vi "SetUpInstruments.vi"(8 "ErrorIn(No Error)":errorcluster caption="entrée d'erreur (pas d'erreur)", 11 "Experiment.lvclass":refnum<class "Experiment.lvclass">) -> (0 "sortie d'erreur":errorcluster, 3 "Experiment.lvclass Out":refnum<class "Experiment.lvclass">)   [LabVIEW 2019, in "Experiment.lvclass"]
uses:
  Experiment.lvclass
  LoadInstr.ctl
  SetUpInstrStates.ctl
  Experiment.lvclass/Experiment.ctl
  DevicesClass/BaseDevice/BaseDevice.lvclass
panel:
  out "Classindex":i32
  in  "ScanRes":bool=TRUE
  in  "Modify":bool
  in  "Remove":bool
  in  "LoadInstr":T1
  in  "LoadedDev":string(tree)
  in  "AvailableDev":string(tree)
  in  "stop":bool
  in  "Add Instrument":bool
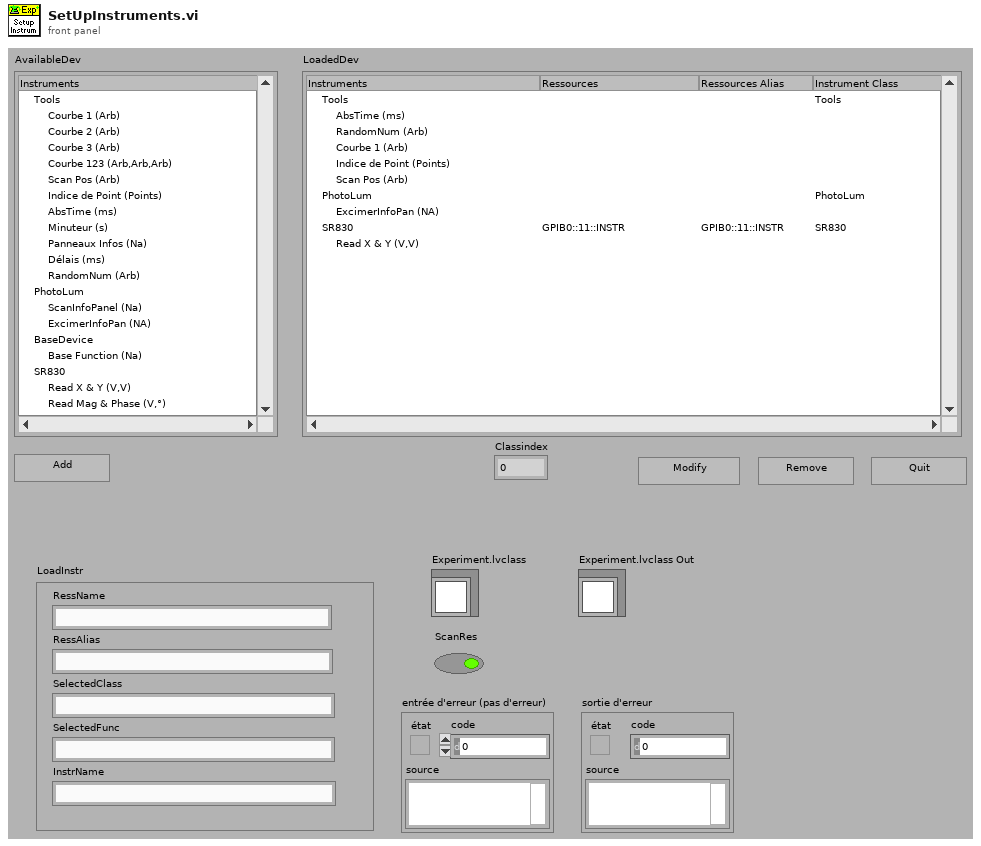
[diagram p1: front panel]
types:
  T1 = typedef "LoadInstr.ctl" = cluster{"SelectedClass":string, "SelectedFunc":string, "InstrName":string, "RessAlias":string, "RessName":string}
  T2 = typedef "SetUpInstrStates.ctl" = enum16{"InitCtrls", "InitProg", "CheckIfInstr", "AddNonInstrFunc", "InstrClassExist?", "AddFuncNewInstr", "AddFuncExInstr", "FuncToWhichInstr?", "ConfirmUnload?", "Unload Instrument", "Unload Function", "ModifyInstr", "Stop", "Error"}
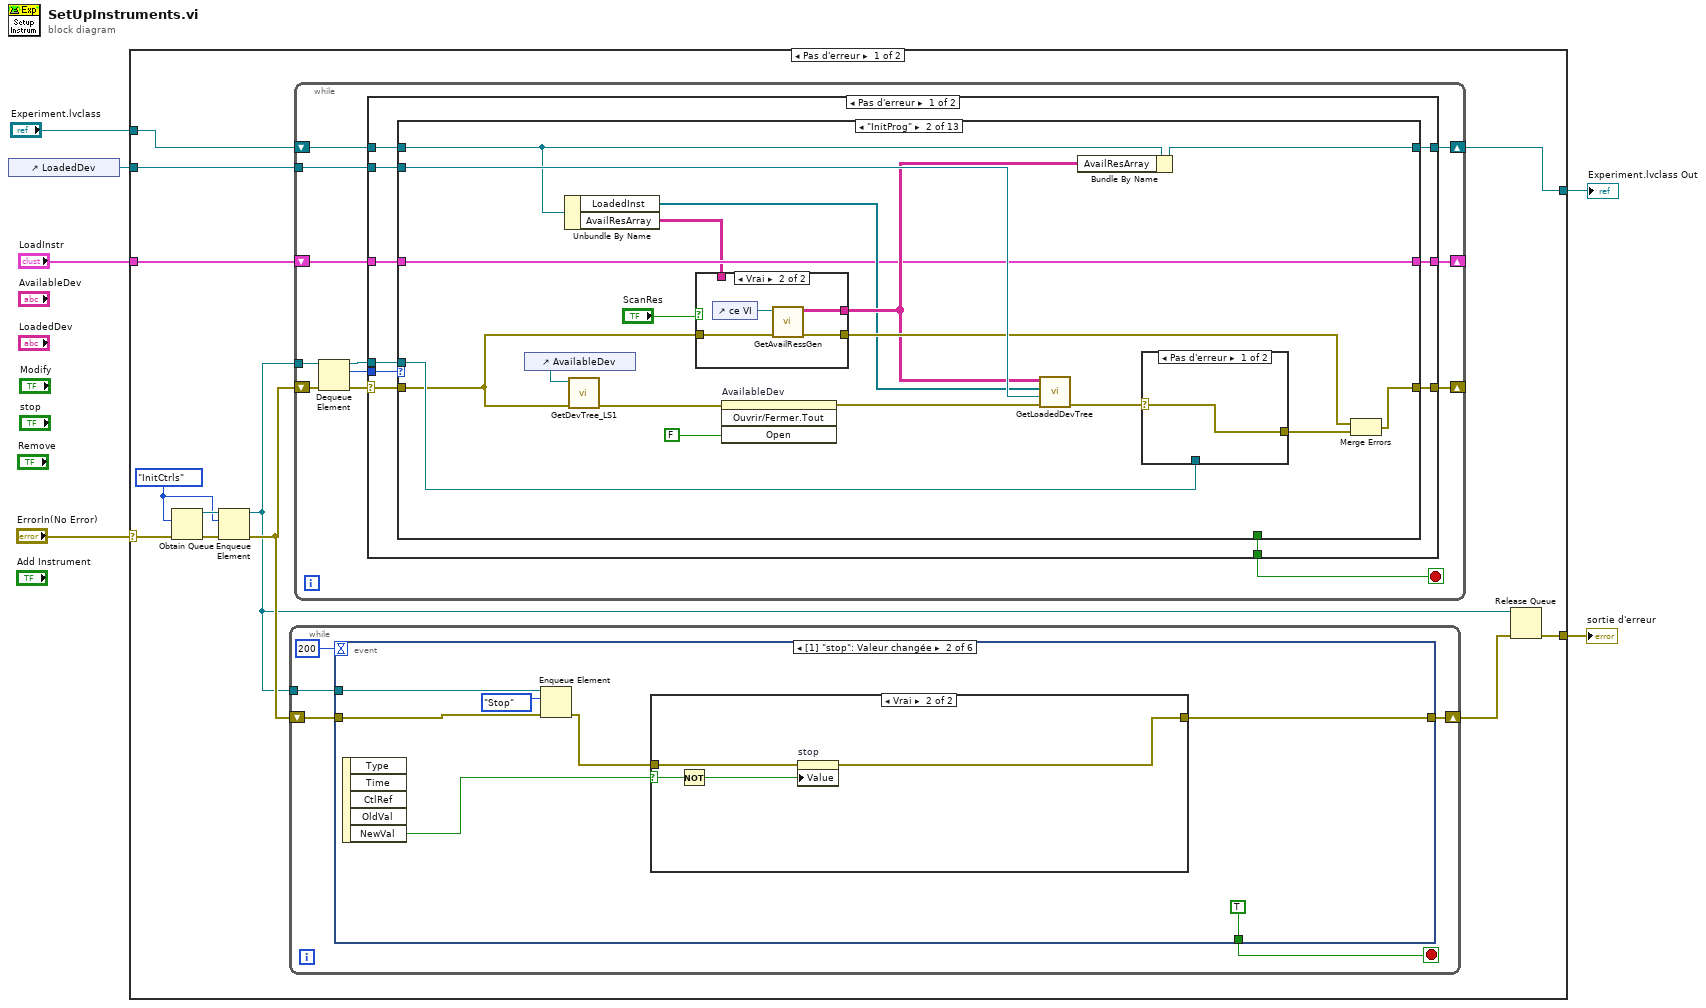
[diagram p0: block diagram]
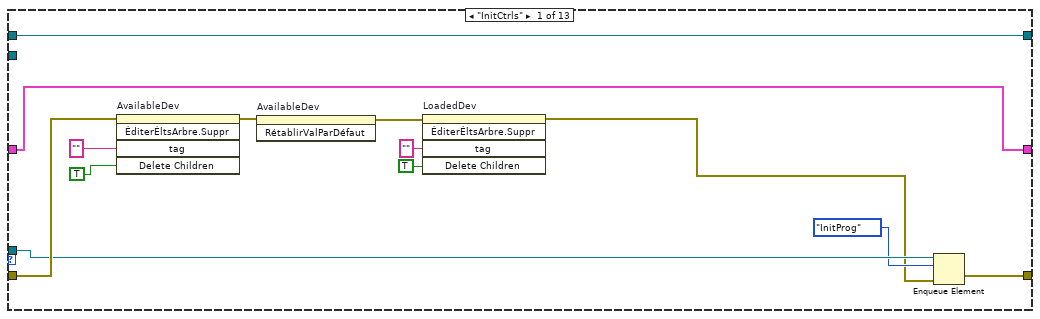
[diagram p2: hidden frame]
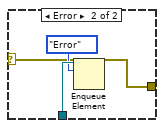
[diagram p4: hidden frame]
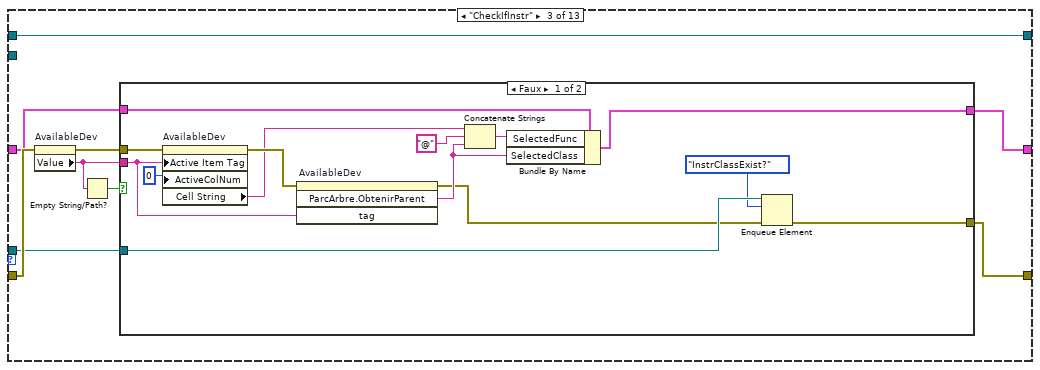
[diagram p5: hidden frame]
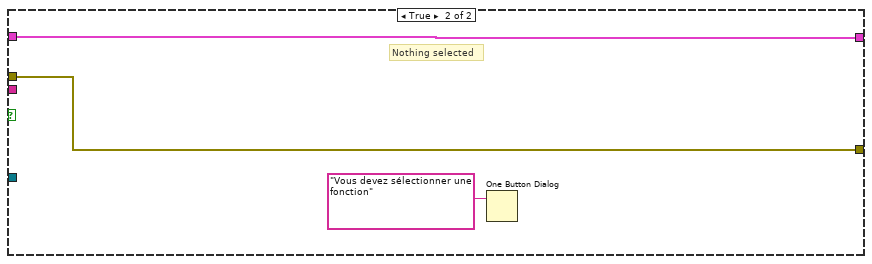
[diagram p6: hidden frame]
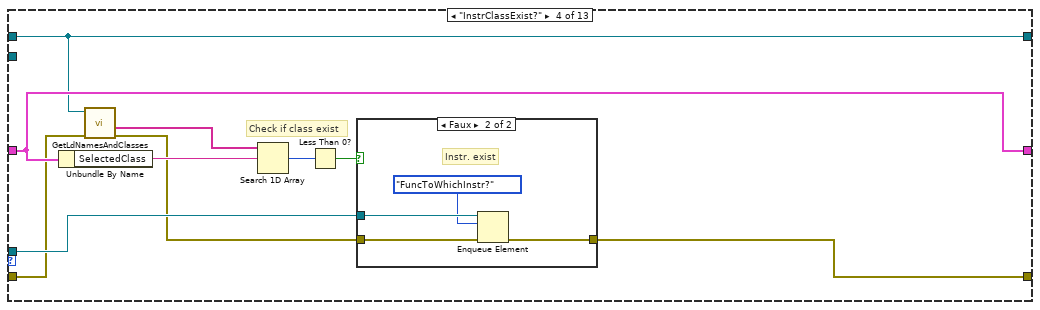
[diagram p7: hidden frame]
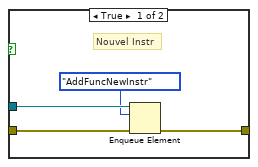
[diagram p8: hidden frame]
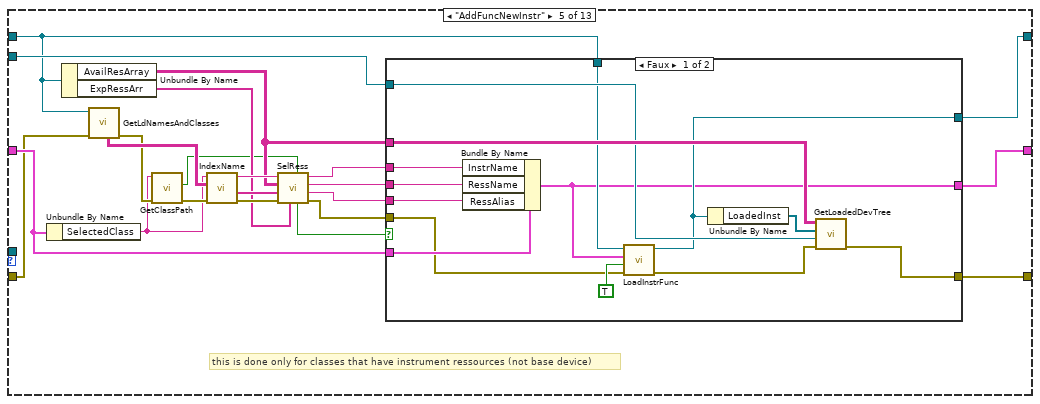
[diagram p9: hidden frame]
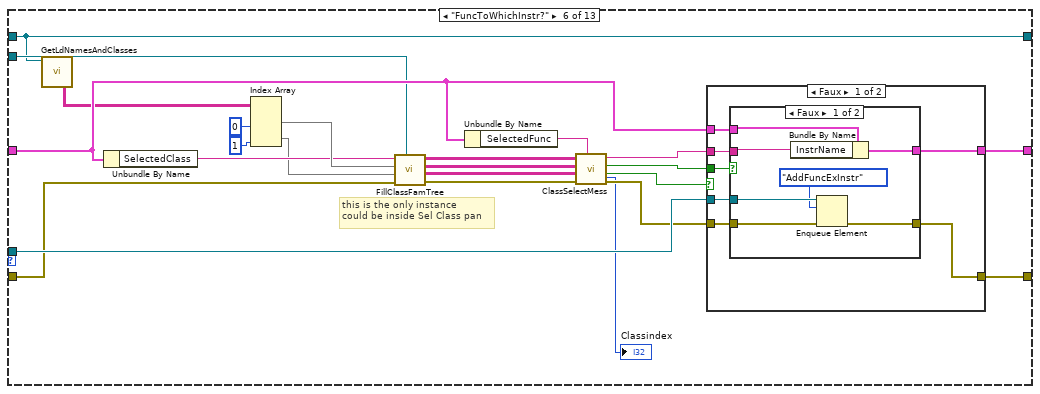
[diagram p11: hidden frame]
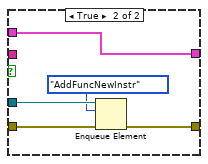
[diagram p12: hidden frame]
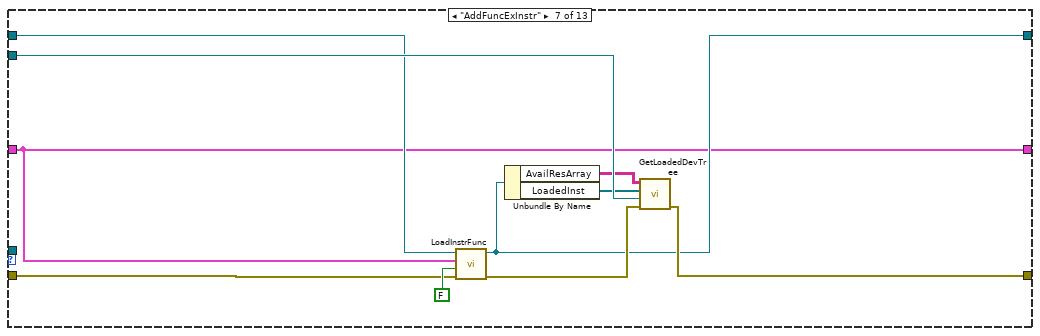
[diagram p14: hidden frame]
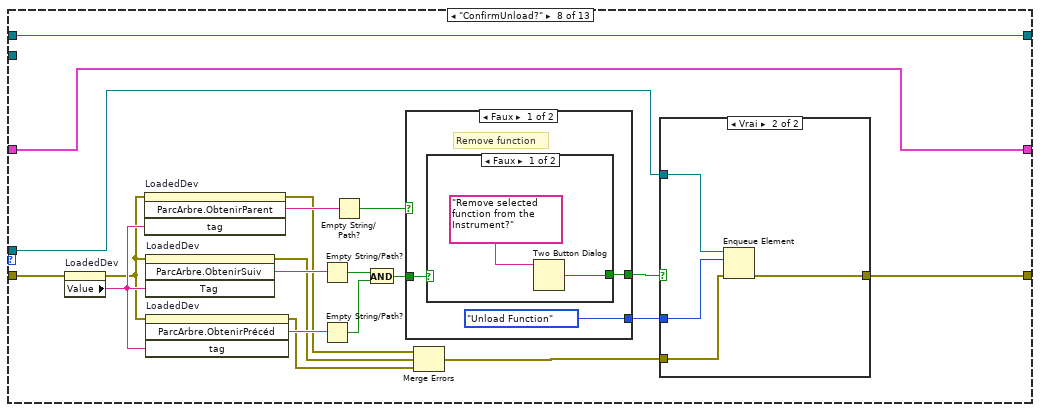
[diagram p15: hidden frame]
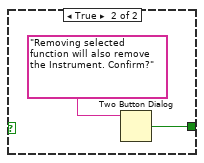
[diagram p17: hidden frame]
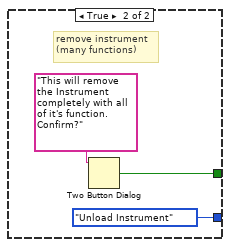
[diagram p18: hidden frame]
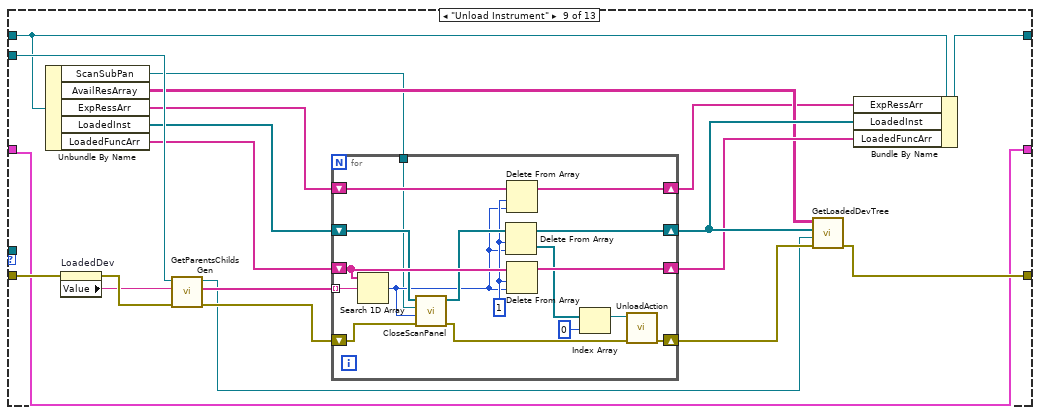
[diagram p19: hidden frame]
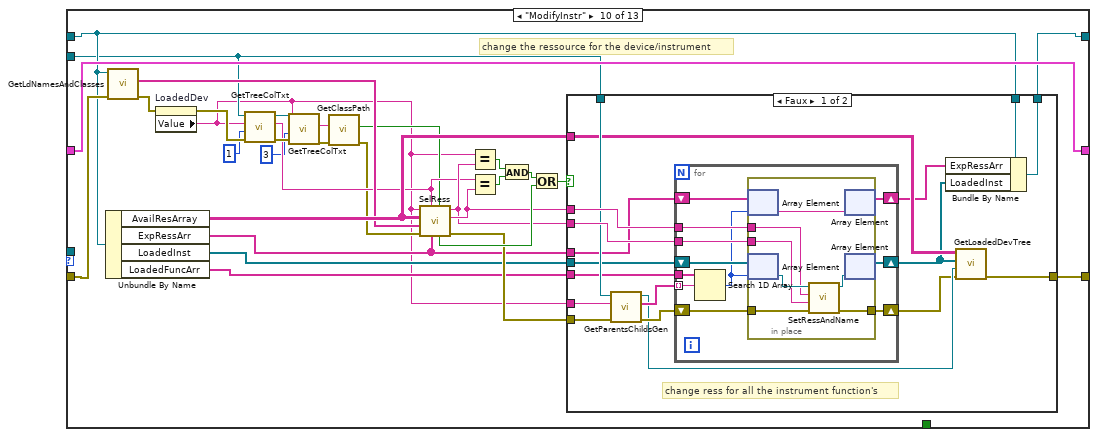
[diagram p20: hidden frame]
diagram:
  n1 = control-ref of="LoadedDev"() -> (w4:refnum<vi>)
  n2 = case shown="Pas d'erreur" "ErrorIn(No Error)" {
    selector: "ErrorIn(No Error)" -> [w9 w479]
    tunnel: "LoadInstr" -> [w14 _]
    tunnel: w4 -> [w13 _]
    tunnel: [w10 w479] -> w3
    tunnel: "Experiment.lvclass" -> [w8 w478]
    tunnel: [w7 w478] -> w1
    frame No Error {
      w16 = SetUpInstrStates."InitCtrls" ("Énum")
      n3 = Obtain Queue(element data type=w16, error in (no error)=w9) -> (queue out=w18:refnum<queue>, error out=w17:errorcluster)  [unwired: 3 in, 1 out]
      n4 = Enqueue Element(queue=w18, element=w16, error in (no error)=w17) -> (queue out=w11:refnum<queue>, error out=w15:errorcluster)  [unwired: 1 in, 1 out]
      n5 = while {
        shift-right: [w397] -> w12
        shift-left: w15 -> [w400]
        tunnel: w11 -> [w398]
        stop <- w399 stop-if-true
        n6 = event shown="[1] \"stop\": Valeur changée" {
          selector: _ -> [_ _ _ _ _ _]
          dyn-events: _ -> [_ _ _ _ _ _]
          timeout: 200 -> [_ _ _ _ _ _]
          tunnel: w400 -> [_ w407 w420 w424 w434 w439]
          tunnel: [_ TRUE ("stop") _ TRUE ("stop") _ _] -> w399
          tunnel: w398 -> [_ w408 w419 w425 w433 w437]
          tunnel: [_ w402 w417 w423 w431 w438] -> w397
          event Timeout {
            n7 = event-data() -> ()  [unwired: 1 in, 2 out]
          }
          event "stop": Value Change {
            n8 = event-data() -> ("NewVal"=w404:bool)  [unwired: 1 in, 4 out]
            n9 = Enqueue Element(queue=w408, element=SetUpInstrStates."Stop" ("élément"), error in (no error)=w407) -> (error out=w403:errorcluster)  [unwired: 1 in, 2 out]
            n10 = case shown="Vrai" w404 {
              selector: w404 -> [_ w413]
              tunnel: w403 -> [w409 w411]
              tunnel: [w409 w410] -> w402
              frame False {
              }
              frame True {
                n11 = Not(x=w413) -> (.not. x?=w412:bool)
                n12 = property on="stop" class="Bool (strict)"(error in=w411, "Value"=w412) -> (error out=w410:errorcluster)  [unwired: 1 in, 1 out]
              }
            }
          }
          event "Add Instrument": Value Change {
            n13 = event-data() -> ("NewVal"=w416:bool)  [unwired: 1 in, 4 out]
            n14 = Wait (ms)(milliseconds to wait=u32 200 ("attente (ms)")) -> (millisecond timer value=w414:u32)
            n15 = Enqueue Element(queue=w419, element=SetUpInstrStates."CheckIfInstr" ("élément"), error in (no error)=w420) -> (error out=w417:errorcluster)  [unwired: 1 in, 2 out]
            n16 = case shown="Vrai" w416 {
              selector: w416 -> [_ w422]
              tunnel: w414 -> [_ _]
              frame False {
              }
              frame True {
                n17 = Not(x=w422) -> (.not. x?=w421:bool)
                n18 = property on="Add Instrument" class="Bool (strict)"("Value"=w421) -> ()  [unwired: 2 in, 2 out]
              }
            }
          }
          event Panel Close {
            n19 = event-data() -> ()  [unwired: 1 in, 4 out]
            n20 = Enqueue Element(queue=w425, element=SetUpInstrStates."Stop" ("élément"), error in (no error)=w424) -> (error out=w423:errorcluster)  [unwired: 1 in, 2 out]
          }
          event "Remove": Value Change {
            n21 = event-data() -> ("NewVal"=w430:bool)  [unwired: 1 in, 4 out]
            n22 = Wait (ms)(milliseconds to wait=u32 200 ("attente (ms)")) -> (millisecond timer value=w428:u32)
            n23 = Enqueue Element(queue=w433, element=SetUpInstrStates."ConfirmUnload?" ("élément"), error in (no error)=w434) -> (error out=w431:errorcluster)  [unwired: 1 in, 2 out]
            n24 = case shown="Vrai" w430 {
              selector: w430 -> [_ w436]
              tunnel: w428 -> [_ _]
              frame False {
              }
              frame True {
                n25 = Not(x=w436) -> (.not. x?=w435:bool)
                n26 = property on="Remove" class="Bool (strict)"("Value"=w435) -> ()  [unwired: 2 in, 2 out]
              }
            }
          }
          event "Modify": Value Change {
            n27 = event-data() -> ("NewVal"=w440:bool)  [unwired: 1 in]
            n28 = case shown="Vrai" w440 {
              tunnel: w439 -> [w441 w447]
              tunnel: [w441 w445] -> w438
              tunnel: w437 -> [_ w443]
              frame False {
              }
              frame True {
                n29 = property on="LoadedDev" class="Arbre (strict)"(error in=w447) -> (error out=w454:errorcluster, "Value"=w442:string)  [unwired: 1 in, 1 out]
                n30 = invoke on="LoadedDev" class="Arbre (strict)" method="ParcArbre.ObtenirEnfant"(error in=w454, "Tag"=w442) -> (error out=w451:errorcluster, "Navigate Tree:Get Child"=w456:string)  [unwired: 2 in, 2 out]
                n31 = invoke on="LoadedDev" class="Arbre (strict)" method="ParcArbre.ObtenirParent"(error in=w454, "tag"=w442) -> (error out=w452:errorcluster, "Navigate Tree:Get Parent"=w453:string)  [unwired: 2 in, 2 out]
                n32 = Merge Errors(w451, w452) -> (w450:errorcluster)
                n33 = Empty String/Path?(string/path=w456) -> (empty?=w455:bool)
                n34 = case shown="Faux" w455 {
                  tunnel: w453 -> [_ w469]
                  tunnel: w450 -> [w463 w464]
                  tunnel: [TRUE w471] -> w449
                  tunnel: [w463 w470] -> w448
                  tunnel: w442 -> [_ _]
                  frame False {
                    # "instrument selected"
                  }
                  frame True {
                    # "func selected"
                    n35 = Format Into String(format string="This will modify parent instrument %s and all of it's functions! Continue? " ("message"), error in=w464, w469) -> (resulting string=w467:string, error out=w466:errorcluster)  [unwired: 1 in]
                    n36 = Two Button Dialog(message=w467) -> (T button?=w465:bool)  [unwired: 2 in]
                    n37 = case shown="Vrai" w465 {
                      selector: w465 -> [w473 w475]
                      tunnel: w469 -> [_ w477]
                      tunnel: w466 -> [w472 w476]
                      tunnel: [w473 w475] -> w471
                      tunnel: [w472 w474] -> w470
                      frame False {
                      }
                      frame True {
                        n38 = property on="LoadedDev" class="Arbre (strict)"(error in=w476, "Value"=w477) -> (error out=w474:errorcluster)  [unwired: 1 in, 1 out]
                      }
                    }
                  }
                }
                n39 = case shown="Vrai" w449 {
                  tunnel: w448 -> [w457 w460]
                  tunnel: [w457 w459] -> w446
                  tunnel: w443 -> [_ w458]
                  frame False {
                  }
                  frame True {
                    n40 = Enqueue Element(queue=w458, element=SetUpInstrStates."ModifyInstr" ("élément"), error in (no error)=w460) -> (error out=w459:errorcluster)  [unwired: 1 in, 2 out]
                  }
                }
                n41 = property on="Modify" class="Bool (strict)"(error in=w446, "Value"=FALSE ("Modify")) -> (error out=w445:errorcluster)  [unwired: 1 in, 1 out]
              }
            }
          }
        }
      }
      n42 = while {
        tunnel: w11 -> [w27]
        shift-right: [w24] -> _
        shift-left: w15 -> [w30]
        shift-right: [w21] -> _
        shift-left: w14 -> [w23]
        tunnel: w13 -> [w22]
        shift-right: [w19] -> w7
        shift-left: w8 -> [w20]
        stop <- w26 stop-if-true
        n43 = Dequeue Element(queue=w27, error in (no error)=w30) -> (queue out=w25:refnum<queue>, element=w28:T2, error out=w29:errorcluster)  [unwired: 1 in, 1 out]
        n44 = case shown="Pas d'erreur" w29 {
          selector: w29 -> [w38 w395]
          tunnel: w28 -> [w40 _]
          tunnel: [w39 FALSE] -> w26
          tunnel: w25 -> [w37 _]
          tunnel: [w36 w391] -> w24
          tunnel: w23 -> [w35 w394]
          tunnel: w22 -> [w34 _]
          tunnel: [w33 w394] -> w21
          tunnel: w20 -> [w32 w393]
          tunnel: [w31 w393] -> w19
          frame No Error {
            n45 = case shown="\"InitProg\"" w40 {
              tunnel: [_ _ _ _ _ _ _ _ _ _ _ TRUE TRUE] -> w39
              tunnel: w38 -> [w50 w56 w90 w109 w130 w175 w211 w238 w273 w307 w382 w384 w388]
              tunnel: w37 -> [w49 w67 w89 w116 _ w181 _ w223 _ _ _ _ _]
              tunnel: [w48 w66 w88 w113 w145 w180 w215 w221 w272 w317 w379 w384 w388] -> w36
              tunnel: w35 -> [w46 w57 w87 w114 w139 w185 w209 w220 w255 w308 w361 w385 w389]
              tunnel: w34 -> [_ w63 _ _ w138 w174 w217 _ w270 w301 w380 _ _]
              tunnel: [w46 w57 w86 w114 w137 w183 w209 w220 w255 w308 w361 w385 w389] -> w33
              tunnel: w32 -> [w45 w59 w85 w111 w131 w167 w214 w219 w265 w305 w373 w383 w387]
              tunnel: [w45 w61 w85 w111 w135 w167 w213 w219 w262 w304 w372 w383 w387] -> w31
              frame "InitCtrls" {
                n46 = invoke on="AvailableDev" class="Arbre (strict)" method="ÉditerÉltsArbre.Suppr"(error in=w50, "tag"="" ("Tag"), "Delete Children"=TRUE ("Supprimer les enfants ?")) -> (error out=w51:errorcluster)  [unwired: 2 in, 4 out]
                n47 = invoke on="AvailableDev" class="Arbre (strict)" method="RétablirValParDéfaut"(error in=w51) -> (error out=w44:errorcluster)  [unwired: 2 in, 2 out]
                n48 = invoke on="LoadedDev" class="Arbre (strict)" method="ÉditerÉltsArbre.Suppr"(error in=w44, "tag"="" ("Tag"), "Delete Children"=TRUE ("Supprimer les enfants ?")) -> (error out=w43:errorcluster)  [unwired: 2 in, 4 out]
                n49 = Enqueue Element(queue=w49, element=SetUpInstrStates."InitProg" ("élément"), error in (no error)=w43) -> (error out=w48:errorcluster)  [unwired: 1 in, 2 out]
              }
              frame "InitProg" {
                n50 = control-ref of="AvailableDev"() -> (w69:refnum<vi>)
                n51 = Unbundle By Name(w59) -> ("LoadedInst"=w58:refnum<class "BaseDevice.lvclass">[], "AvailResArray"=w55:string[][])
                n52 = call "GetDevTree_LS1.vi"("ErrorIn"=w56, "TreeRefIn"=w69) -> ("ErrorOut"=w70:errorcluster)  [unwired: 8 in, 1 out]
                n53 = case shown="Vrai" "ScanRes" {
                  tunnel: [w72 w77] -> w62
                  tunnel: [w73 w76] -> w60
                  tunnel: w56 -> [w72 w75]
                  tunnel: w55 -> [w73 _]
                  frame False {
                  }
                  frame True {
                    n54 = control-ref of="ce VI"() -> (w74:refnum<vi>)
                    n55 = call <userlib>:"GetAvailRessGen.vi"("ErrorIn(No Error)"=w75, "VI reference"=w74) -> ("sortie d'erreur"=w77:errorcluster, "ResArray"=w76:string[][])  [unwired: 8 in]
                  }
                }
                n56 = invoke on="AvailableDev" class="Arbre (strict)" method="Ouvrir/Fermer.Tout"(error in=w70, "Open"=FALSE ("Ouvrir ?")) -> (error out=w71:errorcluster)  [unwired: 2 in, 3 out]
                n57 = call "GetLoadedDevTree.vi"("ErrorIn"=w71, "TreeRefIn"=w63, "LoadedInst"=w58, "AvailRessArray"=w60) -> ("ErrorOut"=w64:errorcluster)  [unwired: 7 in]
                n58 = Bundle By Name(cluster=w59, "AvailResArray"=w60) -> (w61:refnum<class "Experiment.lvclass">)
                n59 = case shown="Pas d'erreur" w64 {
                  selector: w64 -> [w78 w79]
                  tunnel: w67 -> [_ w81]
                  tunnel: [w78 w79] -> w65
                  frame No Error {
                  }
                  frame Error {
                    n60 = Enqueue Element(queue=w81, element=SetUpInstrStates."Error" ("élément")) -> ()  [unwired: 2 in, 3 out]
                  }
                }
                n61 = Merge Errors(w62, w65) -> (w66:errorcluster)
              }
              frame "CheckIfInstr" {
                n62 = property on="AvailableDev" class="Arbre (strict)"(error in=w90) -> (error out=w83:errorcluster, "Value"=w82:string)  [unwired: 1 in, 1 out]
                n63 = Empty String/Path?(string/path=w82) -> (empty?=w84:bool)
                n64 = case shown="Faux" w84 {
                  tunnel: w89 -> [w104 _]
                  tunnel: [w103 w105] -> w88
                  tunnel: w87 -> [w102 w106]
                  tunnel: [w93 w106] -> w86
                  tunnel: w83 -> [w95 w105]
                  tunnel: w82 -> [w94 _]
                  frame False {
                    n65 = property on="AvailableDev" class="Arbre (strict)"(error in=w95, "Active Item Tag"=w94, "ActiveColNum"=0 ("Cellule active : numéro de la colonne active")) -> (error out=w100:errorcluster, "Cell String"=w99:string)  [unwired: 1 in, 1 out]
                    n66 = invoke on="AvailableDev" class="Arbre (strict)" method="ParcArbre.ObtenirParent"(error in=w100, "tag"=w94) -> (error out=w91:errorcluster, "Navigate Tree:Get Parent"=w96:string)  [unwired: 2 in, 2 out]
                    n67 = Concatenate Strings(w99, "@" ("chaîne"), w96) -> (w97:string)
                    n68 = Bundle By Name(cluster=w102, "SelectedFunc"=w97, "SelectedClass"=w96) -> (w93:T1)
                    n69 = Enqueue Element(queue=w104, element=SetUpInstrStates."InstrClassExist?" ("élément"), error in (no error)=w91) -> (error out=w103:errorcluster)  [unwired: 1 in, 2 out]
                  }
                  frame True {
                    # "Nothing selected"
                    n70 = One Button Dialog(message="Vous devez sélectionner une fonction") -> ()  [unwired: 1 in, 1 out]
                  }
                }
              }
              frame "InstrClassExist?" {
                # "Check if class exist"
                n71 = Unbundle By Name(w114) -> ("SelectedClass"=w112:string)
                n72 = call "GetLdNamesAndClasses.vi"("error in (no error)"=w109, "Experiment en entrée"=w111) -> ("error out"=w108:errorcluster, "LdClasses"=w110:string[])  [unwired: 5 in, 3 out]
                n73 = Search 1D Array(1D array=w110, element=w112) -> (index of element=w117:i32)  [unwired: 1 in]
                n74 = Less Than 0?(x=w117) -> (x < 0?=w115:bool)
                n75 = case shown="Faux" w115 {
                  tunnel: w116 -> [w121 w125]
                  tunnel: w108 -> [w119 w123]
                  tunnel: [w118 w122] -> w113
                  frame True {
                    # "Nouvel Instr"
                    n76 = Enqueue Element(queue=w121, element=SetUpInstrStates."AddFuncNewInstr" ("élément"), error in (no error)=w119) -> (error out=w118:errorcluster)  [unwired: 1 in, 2 out]
                  }
                  frame False {
                    # "Instr. exist"
                    n77 = Enqueue Element(queue=w125, element=SetUpInstrStates."FuncToWhichInstr?" ("élément"), error in (no error)=w123) -> (error out=w122:errorcluster)  [unwired: 1 in, 2 out]
                  }
                }
              }
              frame "AddFuncNewInstr" {
                # "this is done only for classes that have instrument ressources (not base device)"
                n78 = Unbundle By Name(w139) -> ("SelectedClass"=w126:string)
                n79 = Unbundle By Name(w131) -> ("AvailResArray"=w133:string[][], "ExpRessArr"=w134:string[])
                n80 = call "GetLdNamesAndClasses.vi"("error in (no error)"=w130, "Experiment en entrée"=w131) -> ("error out"=w129:errorcluster, "LdNamesAndClasses"=w132:string[][])  [unwired: 5 in, 3 out]
                n81 = call "GetClassPath.vi"("error in (no error)"=w129, "ClassName"=w126) -> ("error out"=w128:errorcluster, "IsInstrument"=w127:bool)  [unwired: 7 in, 1 out]
                n82 = call "IndexName.vi"("ErrorIn(No Error)"=w128, "ClassArray"=w132, "ClassName"=w126) -> ("sortie d'erreur"=w143:errorcluster, "AllInstrNamesArr"=w136:string[], "Instrument name"=w142:string)  [unwired: 5 in, 1 out]
                n83 = call "SelRess.vi"("Instr"=w127, "UsedRess"=w134, "ErrorIn(No Error)"=w143, "InstrNames"=w136, "RessArray"=w133, "InstrName"=w142) -> ("sortie d'erreur"=w144:errorcluster, "RessAlias"=w140:string, "RessNameOut"=w147:string, "InstrNameOut"=w146:string, "Cancel Out"=w141:bool)  [unwired: 1 in]
                n84 = case shown="Faux" w141 {
                  tunnel: w147 -> [w157 _]
                  tunnel: w146 -> [w158 _]
                  tunnel: [w153 w164] -> w145
                  tunnel: w144 -> [w159 w164]
                  tunnel: w139 -> [w161 w163]
                  tunnel: w140 -> [w156 _]
                  tunnel: w138 -> [w152 _]
                  tunnel: [w148 w163] -> w137
                  tunnel: w133 -> [w155 _]
                  tunnel: w131 -> [w151 w162]
                  tunnel: [w150 w162] -> w135
                  frame False {
                    n85 = Bundle By Name(cluster=w161, "InstrName"=w158, "RessName"=w157, "RessAlias"=w156) -> (w148:T1)
                    n86 = call "LoadInstrFunc.vi"("ErrorIn(No Error)"=w159, "New Instr"=TRUE, "LoadInstr"=w148, "Experiment.lvclass"=w151) -> ("sortie d'erreur"=w154:errorcluster, "Experiment.lvclass Out"=w150:refnum<class "Experiment.lvclass">)  [unwired: 6 in]
                    n87 = Unbundle By Name(w150) -> ("LoadedInst"=w149:refnum<class "BaseDevice.lvclass">[])
                    n88 = call "GetLoadedDevTree.vi"("ErrorIn"=w154, "TreeRefIn"=w152, "LoadedInst"=w149, "AvailRessArray"=w155) -> ("ErrorOut"=w153:errorcluster)  [unwired: 7 in]
                  }
                  frame True {
                    # "operation canceled"
                  }
                }
              }
              frame "FuncToWhichInstr?" {
                # "this is the only instance\ncould be inside Sel Class pan"
                n89 = call "GetLdNamesAndClasses.vi"("Experiment en entrée"=w167) -> ("LdNamesAndClasses"=w166:string[][])  [unwired: 6 in, 4 out]
                n90 = Unbundle By Name(w185) -> ("SelectedClass"=w177:string)
                n91 = Index Array(array=w166, index (col) #1=0 ("indice désactivé (col)"), index (col) #2=1 ("indice désactivé (col)")) -> (element #1=w178:string[], element #2=w176:string[])  [unwired: 2 in]
                n92 = call "FillClassFamTree.vi"("référence"=w174, "ErrorIn(No Error)"=w175, "LdClassArr"=w176, "LdNameArr"=w178, "SelectedClass"=w177) -> ("sortie d'erreur"=w170:errorcluster, "Text"=w171:string[][], "Functions"=w172:string[][], "Classes"=w173:string[][])  [unwired: 3 in]
                n93 = Unbundle By Name(w185) -> ("SelectedFunc"=w184:string)
                n94 = call "ClassSelectMess.vi"("NewFunction"=w184, "ErrorIn(No Error)"=w170, "Text"=w171, "Functions"=w172, "Classes"=w173) -> ("sortie d'erreur"=w169:errorcluster, "CancelOut"=w168:bool, "New"=w179:bool, "InstrNameOut"=w182:string, "Classindex"=→"Classindex":i32)  [unwired: 2 in]
                n95 = case shown="Faux" w168 {
                  tunnel: w185 -> [w194 w208]
                  tunnel: [w193 w208] -> w183
                  tunnel: w182 -> [w192 _]
                  tunnel: w181 -> [w191 _]
                  tunnel: [w190 w207] -> w180
                  tunnel: w179 -> [w189 _]
                  tunnel: w169 -> [w188 w207]
                  frame False {
                    n96 = case shown="Faux" w189 {
                      tunnel: w194 -> [w201 w206]
                      tunnel: [w200 w206] -> w193
                      tunnel: w192 -> [w199 _]
                      tunnel: w191 -> [w198 w205]
                      tunnel: w188 -> [w195 w204]
                      tunnel: [w197 w203] -> w190
                      frame False {
                        n97 = Bundle By Name(cluster=w201, "InstrName"=w199) -> (w200:T1)
                        n98 = Enqueue Element(queue=w198, element=SetUpInstrStates."AddFuncExInstr" ("élément"), error in (no error)=w195) -> (error out=w197:errorcluster)  [unwired: 1 in, 2 out]
                      }
                      frame True {
                        n99 = Enqueue Element(queue=w205, element=SetUpInstrStates."AddFuncNewInstr" ("élément"), error in (no error)=w204) -> (error out=w203:errorcluster)  [unwired: 1 in, 2 out]
                      }
                    }
                  }
                  frame True {
                    # "operation cancelled"
                  }
                }
              }
              frame "AddFuncExInstr" {
                n100 = call "LoadInstrFunc.vi"("ErrorIn(No Error)"=w211, "New Instr"=FALSE, "LoadInstr"=w209, "Experiment.lvclass"=w214) -> ("sortie d'erreur"=w216:errorcluster, "Experiment.lvclass Out"=w213:refnum<class "Experiment.lvclass">)  [unwired: 6 in]
                n101 = Unbundle By Name(w213) -> ("AvailResArray"=w210:string[][], "LoadedInst"=w212:refnum<class "BaseDevice.lvclass">[])
                n102 = call "GetLoadedDevTree.vi"("ErrorIn"=w216, "TreeRefIn"=w217, "LoadedInst"=w212, "AvailRessArray"=w210) -> ("ErrorOut"=w215:errorcluster)  [unwired: 7 in]
              }
              frame "ConfirmUnload?" {
                n103 = property on="LoadedDev" class="Arbre (strict)"(error in=w238) -> (error out=w234:errorcluster, "Value"=w235:string)  [unwired: 1 in, 1 out]
                n104 = invoke on="LoadedDev" class="Arbre (strict)" method="ParcArbre.ObtenirParent"(error in=w234, "tag"=w235) -> (error out=w228:errorcluster, "Navigate Tree:Get Parent"=w237:string)  [unwired: 2 in, 2 out]
                n105 = invoke on="LoadedDev" class="Arbre (strict)" method="ParcArbre.ObtenirSuiv"(error in=w234, "Tag"=w235) -> (error out=w227:errorcluster, "Navigate Tree:Get Next Item"=w233:string)  [unwired: 2 in, 2 out]
                n106 = invoke on="LoadedDev" class="Arbre (strict)" method="ParcArbre.ObtenirPrécéd"(error in=w234, "tag"=w235) -> (error out=w226:errorcluster, "Navigate Tree:Get Previous"=w232:string)  [unwired: 2 in, 2 out]
                n107 = Empty String/Path?(string/path=w233) -> (empty?=w231:bool)
                n108 = Empty String/Path?(string/path=w232) -> (empty?=w230:bool)
                n109 = Empty String/Path?(string/path=w237) -> (empty?=w236:bool)
                n110 = And(x=w231, y=w230) -> (x .and. y?=w229:bool)
                n111 = case shown="Faux" w236 {
                  tunnel: w229 -> [w246 _]
                  tunnel: [w245 w252] -> w222
                  tunnel: [SetUpInstrStates."Unload Function" ("Énum") SetUpInstrStates."Unload Instrument" ("élément")] -> w224
                  frame False {
                    # "Remove function"
                    n112 = case shown="Faux" w246 {
                      tunnel: [w247 w249] -> w245
                      frame False {
                        n113 = Two Button Dialog(message="Remove selected function from the Instrument?") -> (T button?=w247:bool)  [unwired: 2 in]
                      }
                      frame True {
                        n114 = Two Button Dialog(message="Removing selected function will also remove the Instrument. Confirm?") -> (T button?=w249:bool)  [unwired: 2 in]
                      }
                    }
                  }
                  frame True {
                    # "remove instrument\n(many functions)"
                    n115 = Two Button Dialog(message="This will remove the Instrument completely with all of it's function. Confirm?") -> (T button?=w252:bool)  [unwired: 2 in]
                  }
                }
                n116 = Merge Errors(w228, w227, w226) -> (w225:errorcluster)
                n117 = case shown="Vrai" w222 {
                  tunnel: w225 -> [w239 w241]
                  tunnel: w224 -> [_ w242]
                  tunnel: w223 -> [_ w243]
                  tunnel: [w239 w240] -> w221
                  frame False {
                  }
                  frame True {
                    n118 = Enqueue Element(queue=w243, element=w242, error in (no error)=w241) -> (error out=w240:errorcluster)  [unwired: 1 in, 2 out]
                  }
                }
              }
              frame "Unload Instrument" {
                n119 = Unbundle By Name(w265) -> ("ScanSubPan"=w254:refnum<vi>, "AvailResArray"=w258:string[][], "ExpRessArr"=w259:string[], "LoadedInst"=w263:refnum<class "BaseDevice.lvclass">[], "LoadedFuncArr"=w264:string[])
                n120 = property on="LoadedDev" class="Arbre (strict)"(error in=w273) -> (error out=w271:errorcluster, "Value"=w269:string)  [unwired: 1 in, 1 out]
                n121 = call <userlib>:"GetParentsChildsGen.vi"("ErrorIn(No Error)"=w271, "ParentTag"=w269, "TreeRef"=w270) -> ("sortie d'erreur"=w267:errorcluster, "Childs"=w268:string[], "TreeRef Out"=w256:refnum<vi>)  [unwired: 6 in]
                n122 = for {
                  tunnel: w268 -> [w290] mode=indexing
                  shift-right: [w288] -> w260
                  shift-left: w264 -> [w289]
                  shift-right: [w280] -> w261
                  shift-left: w263 -> [w283]
                  shift-right: [w284] -> w266
                  shift-left: w267 -> [w282]
                  shift-right: [w275] -> w257
                  shift-left: w259 -> [w276]
                  tunnel: w254 -> [w274]
                  w278 = 1 ("longueur")
                  n123 = Search 1D Array(1D array=w289, element=w290) -> (index of element=w277:i32)  [unwired: 1 in]
                  n124 = call "CloseScanPanel.vi"("error in (no error)"=w282, "Index"=w277, "SubPanRef"=w274, "LoadedInst"=w283) -> ("sortie d'erreur"=w281:errorcluster, "LoadedInst Out"=w279:refnum<class "BaseDevice.lvclass">[])  [unwired: 6 in]
                  n125 = Delete From Array(array=w279, length=w278, index=w277) -> (deleted portion=w287:refnum<class "BaseDevice.lvclass">[], array with subset deleted=w280:refnum<class "BaseDevice.lvclass">[])
                  n126 = Delete From Array(array=w276, length=w278, index=w277) -> (array with subset deleted=w275:string[])  [unwired: 1 out]
                  n127 = Delete From Array(array=w289, length=w278, index=w277) -> (array with subset deleted=w288:string[])  [unwired: 1 out]
                  n128 = Index Array(array=w287, index=0 ("indice")) -> (element=w286:refnum<class "BaseDevice.lvclass">)
                  n129 = call-dynamic "UnloadAction.vi"("error in (no error)"=w281, "Device en entrée"=w286) -> ("error out"=w284:errorcluster)  [unwired: 8 in, 1 out]
                }
                n130 = call "GetLoadedDevTree.vi"("ErrorIn"=w266, "TreeRefIn"=w256, "LoadedInst"=w261, "AvailRessArray"=w258) -> ("ErrorOut"=w272:errorcluster)  [unwired: 7 in]
                n131 = Bundle By Name(cluster=w265, "ExpRessArr"=w257, "LoadedInst"=w261, "LoadedFuncArr"=w260) -> (w262:refnum<class "Experiment.lvclass">)
              }
              frame "ModifyInstr" {
                # "change the ressource for the device/instrument"
                n132 = Unbundle By Name(w305) -> ("AvailResArray"=w310:string[][], "ExpRessArr"=w309:string[], "LoadedInst"=w311:refnum<class "BaseDevice.lvclass">[], "LoadedFuncArr"=w312:string[])
                n133 = call "GetLdNamesAndClasses.vi"("error in (no error)"=w307, "Experiment en entrée"=w305) -> ("error out"=w306:errorcluster, "LdNames"=w303:string[])  [unwired: 5 in, 3 out]
                n134 = property on="LoadedDev" class="Arbre (strict)"(error in=w306) -> (error out=w302:errorcluster, "Value"=w291:string)  [unwired: 1 in, 1 out]
                n135 = call <userlib>:"GetTreeColTxt.vi"("ErrorIn(No Error)"=w302, "Column"=1, "CellTag"=w291, "TreeRef"=w301) -> ("sortie d'erreur"=w300:errorcluster, "Cellule active : chaîne"=w297:string, "TreeRef"=w299:refnum<vi>)  [unwired: 5 in]
                n136 = call <userlib>:"GetTreeColTxt.vi"("ErrorIn(No Error)"=w300, "Column"=3, "CellTag"=w291, "TreeRef"=w299) -> ("sortie d'erreur"=w294:errorcluster, "Cellule active : chaîne"=w295:string)  [unwired: 5 in, 1 out]
                n137 = call "GetClassPath.vi"("error in (no error)"=w294, "ClassName"=w295) -> ("error out"=w293:errorcluster, "IsInstrument"=w292:bool)  [unwired: 7 in, 1 out]
                n138 = call "SelRess.vi"("Instr"=w292, "UsedRess"=w309, "RessName"=w297, "ErrorIn(No Error)"=w293, "InstrNames"=w303, "RessArray"=w310, "InstrName"=w291) -> ("sortie d'erreur"=w313:errorcluster, "RessNameOut"=w316:string, "InstrNameOut"=w315:string, "Cancel Out"=w318:bool)  [unwired: 1 out]
                n139 = Equal?(x=w291, y=w315) -> (x = y?=w320:bool)
                n140 = Equal?(x=w297, y=w316) -> (x = y?=w321:bool)
                n141 = And(x=w320, y=w321) -> (x .and. y?=w319:bool)
                n142 = Or(x=w319, y=w318) -> (x .or. y?=w314:bool)
                n143 = case shown="Faux" w314 {
                  tunnel: [w330 w359] -> w317
                  tunnel: w316 -> [w339 _]
                  tunnel: w315 -> [w338 _]
                  tunnel: w310 -> [w326 _]
                  tunnel: w301 -> [w333 _]
                  tunnel: w313 -> [w335 w359]
                  tunnel: w291 -> [w334 _]
                  tunnel: w312 -> [w329 _]
                  tunnel: w311 -> [w328 _]
                  tunnel: w309 -> [w327 _]
                  tunnel: w305 -> [w325 w358]
                  tunnel: [w324 w358] -> w304
                  frame False {
                    # "change ress for all the instrument function's"
                    n144 = call <userlib>:"GetParentsChildsGen.vi"("ErrorIn(No Error)"=w335, "ParentTag"=w334, "TreeRef"=w333) -> ("sortie d'erreur"=w336:errorcluster, "Childs"=w337:string[], "TreeRef Out"=w332:refnum<vi>)  [unwired: 6 in]
                    n145 = for {
                      tunnel: w337 -> [w350] mode=indexing
                      tunnel: w329 -> [w349]
                      shift-right: [w346] -> w331
                      shift-left: w336 -> [w347]
                      tunnel: w339 -> [w345]
                      tunnel: w338 -> [w344]
                      shift-right: [w348] -> w322
                      shift-left: w328 -> [w343]
                      shift-right: [w341] -> w323
                      shift-left: w327 -> [w342]
                      n146 = Search 1D Array(1D array=w349, element=w350) -> (index of element=w340:i32)  [unwired: 1 in]
                      n147 = in-place {
                        in-place-border: w347 -> [w357]
                        in-place-border: [w356] -> w346
                        in-place-border: w345 -> [w353]
                        in-place-border: w344 -> [w352]
                        n148 = in-place-array #1(w342, w340) -> (w351:string)
                        n149 = in-place-array #2(w343, w340) -> (w355:refnum<class "BaseDevice.lvclass">)
                        n150 = call "SetRessAndName.vi"("error in (no error)"=w357, "InstrumentName"=w352, "Nom de ressource VISA"=w353, "BaseDevice en entrée"=w355) -> ("error out"=w356:errorcluster, "BaseDevice en sortie"=w354:refnum<class "BaseDevice.lvclass">)  [unwired: 6 in]
                        n151 = in-place-array #1(w351) -> (w341:string[])  [unwired: 1 out]
                        n152 = in-place-array #2(w354) -> (w348:refnum<class "BaseDevice.lvclass">[])  [unwired: 1 out]
                      }
                    }
                    n153 = Bundle By Name(cluster=w325, "ExpRessArr"=w323, "LoadedInst"=w322) -> (w324:refnum<class "Experiment.lvclass">)
                    n154 = call "GetLoadedDevTree.vi"("ErrorIn"=w331, "TreeRefIn"=w332, "LoadedInst"=w322, "AvailRessArray"=w326) -> ("ErrorOut"=w330:errorcluster)  [unwired: 7 in]
                  }
                  frame True {
                    # "No change or cancel"
                  }
                }
              }
              frame "Unload Function" {
                w369 = 1 ("longueur")
                n155 = property on="LoadedDev" class="Arbre (strict)"(error in=w382) -> (error out=w376:errorcluster, "Value"=w381:string)  [unwired: 1 in, 1 out]
                n156 = Unbundle By Name(w373) -> ("ScanSubPan"=w360:refnum<vi>, "ExpRessArr"=w370:string[], "AvailResArray"=w371:string[][], "LoadedInst"=w367:refnum<class "BaseDevice.lvclass">[], "LoadedFuncArr"=w366:string[])
                n157 = Search 1D Array(1D array=w366, element=w381) -> (index of element=w368:i32)  [unwired: 1 in]
                n158 = call "CloseScanPanel.vi"("error in (no error)"=w376, "Index"=w368, "SubPanRef"=w360, "LoadedInst"=w367) -> ("sortie d'erreur"=w375:errorcluster, "LoadedInst Out"=w374:refnum<class "BaseDevice.lvclass">[])  [unwired: 6 in]
                n159 = Delete From Array(array=w374, length=w369, index=w368) -> (deleted portion=w378:refnum<class "BaseDevice.lvclass">[], array with subset deleted=w364:refnum<class "BaseDevice.lvclass">[])
                n160 = Delete From Array(array=w366, length=w369, index=w368) -> (array with subset deleted=w365:string[])  [unwired: 1 out]
                n161 = Delete From Array(array=w370, length=w369, index=w368) -> (array with subset deleted=w363:string[])  [unwired: 1 out]
                n162 = Index Array(array=w378) -> (element=w362:refnum<class "BaseDevice.lvclass">)  [unwired: 1 in]
                n163 = call-dynamic "UnloadAction.vi"("error in (no error)"=w375, "Device en entrée"=w362) -> ("error out"=w377:errorcluster)  [unwired: 8 in, 1 out]
                n164 = Bundle By Name(cluster=w373, "ExpRessArr"=w363, "LoadedFuncArr"=w365, "LoadedInst"=w364) -> (w372:refnum<class "Experiment.lvclass">)
                n165 = call "GetLoadedDevTree.vi"("ErrorIn"=w377, "TreeRefIn"=w380, "LoadedInst"=w364, "AvailRessArray"=w371) -> ("ErrorOut"=w379:errorcluster)  [unwired: 7 in]
              }
              frame "Stop" {
              }
              frame "Error", Default {
              }
            }
          }
          frame Error {
            n166 = call <vilib>:"General Error Handler.vi"("error in (no error)"=w395) -> ("error out"=w392:errorcluster)  [unwired: 10 in, 4 out]
            n167 = call <vilib>:"Clear Errors.vi"("error in (no error)"=w392) -> ("error out"=w391:errorcluster)  [unwired: 5 in, 1 out]
          }
        }
      }
      n168 = Release Queue(queue=w11, error in (no error)=w12) -> (error out=w10:errorcluster)  [unwired: 1 in, 2 out]
    }
    frame Error {
    }
  }
  "sortie d'erreur" <- w3
  "Experiment.lvclass Out" <- w1
